vi "Get Engine.vi"(8 "error in (no error)":errorcluster, 11 "SequenceFile in":refnum<class "SequenceFile.lvclass">) -> (0 "error out":errorcluster, 2 "Engine":T1, 3 "SequenceFile out":refnum<class "SequenceFile.lvclass">)   [LabVIEW 2020, in "TSS.lvlib" / "SequenceFile.lvclass"]
uses:
  SequenceFile.lvclass
  Engine/Typedefs/Session Handle.ctl
  Engine/Engine.lvclass
  SequenceFile.lvclass/SequenceFile.ctl
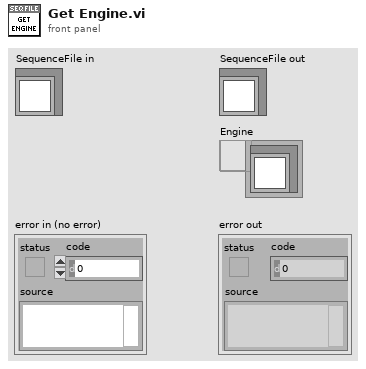
[diagram p1: front panel]
types:
  T1 = typedef "TSS.lvlib/Engine.lvclass/Session Handle.ctl" = refnum<data-value>
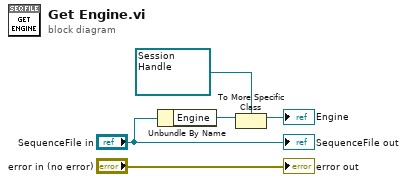
[diagram p0: block diagram]
diagram:
  n1 = Unbundle By Name("SequenceFile in") -> ("Engine"=w3:refnum<data-value>)
  n2 = To More Specific Class(target class=T1 refnum ("Engine"), reference=w3) -> (specific class reference=→"Engine":T1)  [unwired: 1 in, 1 out]
  "error out" <- "error in (no error)"
  "SequenceFile out" <- "SequenceFile in"
